vi "Create Sequence.vi"(6 "Sequence Type (0: Pseudo Random Bit Sequence)":i32(ring) items=["Pseudo Random Bit Sequence", "Clock Pattern Sequence"], 7 "Sequence Length (0)":i32, 8 "error in (no error)":errorcluster, 9 "Clock Pattern Rate (0)":i32, 10 "Polynomial Length (7: Length 7)":i32(ring) items=["Length 7", "Length 9", "Length 11", "Length 15", "Length 23", "Length 31"], 11 "VISA resource name":refnum<visa-resource-name>) -> (0 "error out":errorcluster, 3 "VISA resource name out":refnum<visa-resource-name>)   [LabVIEW 2009, in "Agilent 81150.lvlib"]
doc: "Creates a PRBS (pseudo random bit sequence) or a clock pattern sequence.\n\n<B>Note(s):</B>\nPattern mode must be turned on to use this VI."
uses:
  Agilent 81150.lvlib
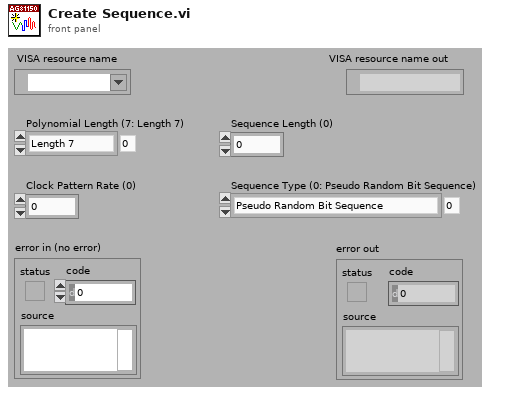
[diagram p1: front panel]
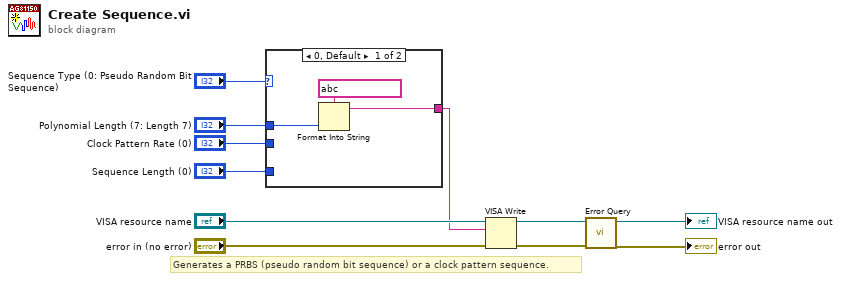
[diagram p0: block diagram]
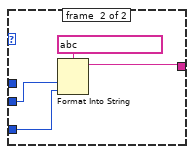
[diagram p2: hidden frame]
diagram:
  # "Generates a PRBS (pseudo random bit sequence) or a clock pattern sequence."
  n1 = case shown="0, Default" "Sequence Type (0: Pseudo Random Bit Sequence)" {
    tunnel: "Polynomial Length (7: Length 7)" -> [w13 _]
    tunnel: [w12 w17] -> w1
    tunnel: "Clock Pattern Rate (0)" -> [_ w16]
    tunnel: "Sequence Length (0)" -> [_ w15]
    frame #0 {
      n2 = Format Into String(format string=string ?, w13) -> (resulting string=w12:string)  [unwired: 2 in, 1 out]
    }
    frame #1 {
      n3 = Format Into String(format string=string ?, w16, w15) -> (resulting string=w17:string)  [unwired: 2 in, 1 out]
    }
  }
  n4 = VISA Write(VISA resource name="VISA resource name", write buffer=w1, error in (no error)="error in (no error)") -> (VISA resource name out=w9:refnum<visa-resource-name>, error out=w8:errorcluster)  [unwired: 1 out]
  n5 = call "Error Query.vi"("error in (no error)"=w8, "VISA resource name"=w9) -> ("error out"=→"error out":errorcluster, "VISA resource name out"=→"VISA resource name out":refnum<visa-resource-name>)  [unwired: 6 in, 2 out]
